vi "Avg4Samps.vi"(2 "Input":i16[](array[numeric])=[0, 0], 3 "Start":bool=TRUE) -> (16 "OuputAvg":i16, 17 "Output Valid":bool)   [LabVIEW 2015]
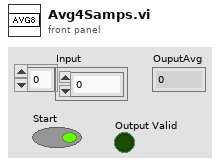
[diagram p1: front panel]
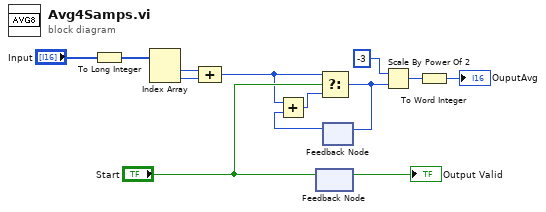
[diagram p0: block diagram]
diagram:
  n1 = To Long Integer(number="Input") -> (32bit integer=w2:i32[])
  n2 = Index Array(array=w2) -> (element #1=w4:i32, element #2=w3:i32)  [unwired: 2 in]
  n3 = Compound Arithmetic op=ADD(w4, w3) -> (w1:i32)
  n4 = feedback #1() -> (→"Output Valid":bool)  [unwired: 1 in]
  n5 = feedback-in #1("Start") -> ()
  n6 = feedback #2() -> (w9:i32)  [unwired: 1 in]
  n7 = Add(x=w1, y=w9) -> (x+y=w10:i32)
  n8 = Select(t=w1, s="Start", f=w10) -> (s? t:f=w8:i32)
  n9 = feedback-in #2(w8) -> ()
  n10 = Scale By Power Of 2(n=i16 -3, x=w8) -> (x*2^n=w12:i32)
  n11 = To Word Integer(number=w12) -> (16bit integer=→"OuputAvg":i16)
